vi "add channel to assembly dialog.vi"(6 "user event":T1, 8 "error in":errorcluster, 9 "channel list":refnum<vi>, 10 "engine configuration in":refnum<class "engine configuration.lvclass">, 11 "EthernetIP configuration in":refnum<class "EthernetIP configuration.lvclass">) -> (0 "error out":errorcluster, 2 "engine configuration out":refnum<class "engine configuration.lvclass">, 3 "EthernetIP configuration out":refnum<class "EthernetIP configuration.lvclass">)   [LabVIEW 2013, in "EthernetIP editor node.lvclass"]
uses:
  EthernetIP editor node.lvclass
  <vilib>/CEF_TreeControl/Controls/EventCluster.ctl
  <vilib>/CEF_TreeControl/NISE_CEF_TreeControl.lvlib
  <vilib>/NI/TBM Modules/Ethernet IP/configuration/EthernetIP configuration.lvclass
  <vilib>/NI/Module Execution Interface/Engine Configuration/engine configuration.lvclass
  <vilib>/NI/TBM Modules/Ethernet IP/channel/EthernetIP Channel.lvclass
  <vilib>/NI/Tag Bus Module Framework/root configuration/TBM configuration.lvclass
  <vilib>/CEF_TreeControl/Node/UserEventRef.ctl
  <vilib>/CEF_TreeControl/Node/NISE_CEF_Node.lvclass
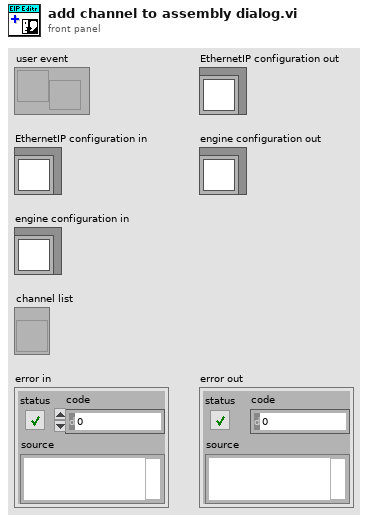
[diagram p1: front panel]
types:
  T1 = typedef "NISE_CEF_Node.lvclass/UserEventRef.ctl" = refnum<user-event>
  T2 = typedef "EthernetIP configuration.lvclass/assembly definition.ctl" = cluster{"name":string, "Instance ID":u32, "Type":T3, "Size (elements)":u32, "big endian?":bool, "data type":T4}
  T3 = typedef "EthernetIP configuration.lvclass/assembly type.ctl" = enum32{"Producing", "Consuming"}
  T4 = typedef "tag bus.lvlib/tag descriptor.lvclass/Data Type.ctl" = enum16{"Double", "Single", "I64", "I32", "I16", "I8", "U64", "U32", "U16", "U8", "Boolean", "String", "Array of Double", "Array of Single", "Array of I64", "Array of I32", "Array of I16", "Array of I8", "Array of U64", "Array of U32", "Array of U16", "Array of U8", "Array of Boolean", "Array of String"}
  T5 = typedef "NISE_CEF_TreeControl.lvlib/EventCluster.ctl" = cluster{"command":string, "data":string}
  T6 = typedef "EthernetIP editor node.lvclass/table line.ctl" = cluster{"eip channels":refnum<class "EthernetIP Channel.lvclass">, "tag name":string}
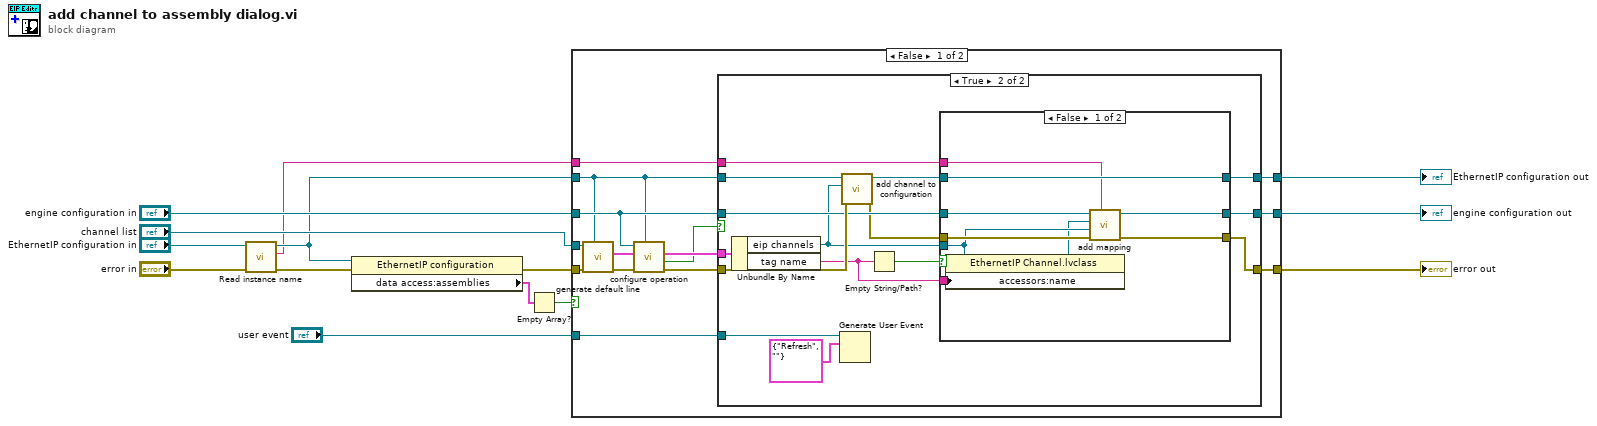
[diagram p0: block diagram]
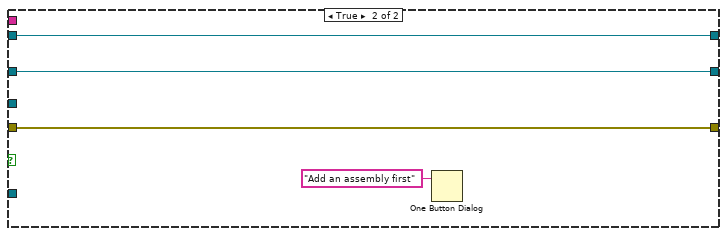
[diagram p4: hidden frame]
diagram:
  n1 = call <vilib>:"Read instance name.vi"("error in"="error in", "configuration in"="EthernetIP configuration in") -> ("error out"=w4:errorcluster, "instance id"=w1:string, "configuration out"=w2:refnum<class "EthernetIP configuration.lvclass">)  [unwired: 7 in]
  n2 = property class="EthernetIP configuration"(reference=w2, error in=w4) -> (error out=w10:errorcluster, "data access:assemblies"=w11:T2[])  [unwired: 1 out]
  n3 = Empty Array?(array=w11) -> (empty?=w9:bool)
  n4 = case shown="False" w9 {
    tunnel: [w28 w61] -> w5
    tunnel: w10 -> [w27 w61]
    tunnel: "channel list" -> [w26 _]
    tunnel: w2 -> [w16 w59]
    tunnel: "engine configuration in" -> [w17 w60]
    tunnel: [w21 w60] -> w14
    tunnel: [w20 w59] -> w13
    tunnel: "user event" -> [w18 _]
    tunnel: w1 -> [w15 _]
    frame False {
      n5 = call "generate default line.vi"("EthernetIP configuration"=w16, "error in"=w27, "operations table"=w26) -> ("error out"=w24:errorcluster, "line"=w25:T6)  [unwired: 7 in]
      n6 = call "configure operation.vi"("EthernetIP configuration"=w16, "error in"=w24, "line item in"=w25, "engine configuration in"=w17) -> ("error out"=w22:errorcluster, "success"=w19:bool, "line item out"=w23:T6)  [unwired: 4 in, 1 out]
      n7 = case shown="True" w19 {
        tunnel: [w31 w35] -> w28
        tunnel: w22 -> [w31 w44]
        tunnel: w17 -> [w30 w42]
        tunnel: w23 -> [_ w45]
        tunnel: w16 -> [w29 w46]
        tunnel: [w30 w41] -> w21
        tunnel: [w29 w36] -> w20
        tunnel: w18 -> [_ w34]
        tunnel: w15 -> [_ w32]
        frame False {
        }
        frame True {
          n8 = Unbundle By Name(w45) -> ("eip channels"=w39:refnum<class "EthernetIP Channel.lvclass">, "tag name"=w38:string)
          n9 = Generate User Event(user event=w34, event data cluster=T5 {"command"="Refresh", "data"=""} ("event data")) -> ()  [unwired: 2 in, 2 out]
          n10 = call <vilib>:"add channel to configuration.vi"("error in"=w44, "TBM channel in"=w39, "EthernetIP configuration in"=w46) -> ("error out"=w40:errorcluster, "EthernetIP configuration out"=w37:refnum<class "EthernetIP configuration.lvclass">)  [unwired: 7 in]
          n11 = Empty String/Path?(string/path=w38) -> (empty?=w43:bool)
          n12 = case shown="False" w43 {
            tunnel: w42 -> [w55 w58]
            tunnel: [w54 w58] -> w41
            tunnel: w40 -> [w53 w57]
            tunnel: w39 -> [w52 _]
            tunnel: w38 -> [w51 _]
            tunnel: [w49 w57] -> w35
            tunnel: w37 -> [w48 w56]
            tunnel: [w48 w56] -> w36
            tunnel: w32 -> [w47 _]
            frame False {
              n13 = property class="EthernetIP Channel.lvclass"(reference=w52, "accessors:name"=w51) -> (reference out=w50:refnum<class "EthernetIP Channel.lvclass">)  [unwired: 1 in, 1 out]
              n14 = call <vilib>:"add mapping.vi"("owner ID"=w47, "error in"=w53, "channel"=w52, "tag descriptor"=w50, "engine configuration"=w55) -> ("error out"=w49:errorcluster, "engine configuration out"=w54:refnum<class "engine configuration.lvclass">)  [unwired: 5 in]
            }
            frame True {
            }
          }
        }
      }
    }
    frame True {
      n15 = One Button Dialog(message="Add an assembly first") -> ()  [unwired: 1 in, 1 out]
    }
  }
  "engine configuration out" <- w14
  "EthernetIP configuration out" <- w13
  "error out" <- w5
